vi "adam-analog-data-read.vi"(8 "error in (no error)":errorcluster, 9 "overwrite-command":string, 10 "current-buffer":string, 11 "VISA Refnum in":refnum<visa-resource-name>) -> (0 "error out":errorcluster, 1 "return count":u32, 2 "read buffer":string, 3 "VISA Refnum Out":refnum<visa-resource-name>, 5 "Bytes at Port":u32)   [LabVIEW 2024]
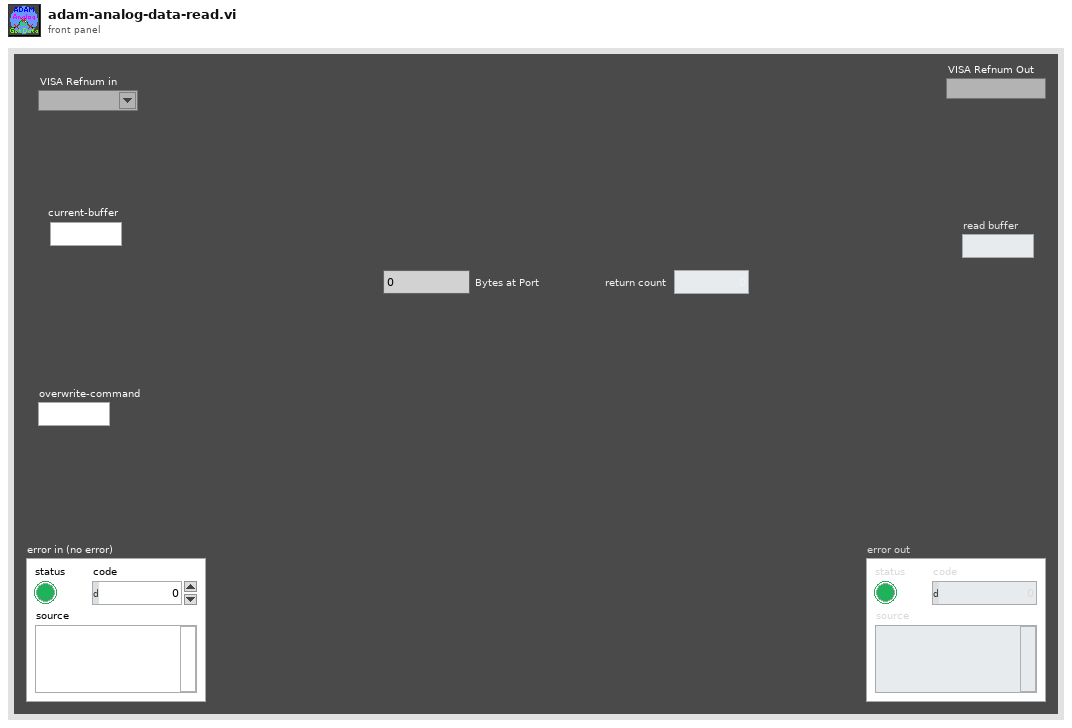
[diagram p1: front panel]
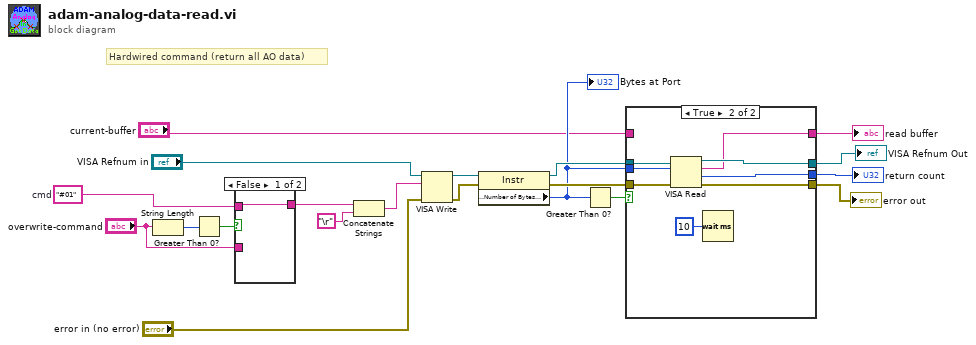
[diagram p0: block diagram]
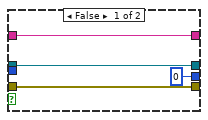
[diagram p3: hidden frame]
diagram:
  w12 = "#01"  # cmd
  # "Hardwired command (return all AO data)"
  n1 = String Length(string="overwrite-command") -> (length=w15:i32)
  n2 = Greater Than 0?(x=w15) -> (x > 0?=w14:bool)
  n3 = case shown="False" w14 {
    tunnel: "overwrite-command" -> [_ w22]
    tunnel: w12 -> [w21 _]
    tunnel: [w21 w22] -> w2
    frame False {
    }
    frame True {
    }
  }
  n4 = Concatenate Strings(w2, "\r") -> (w3:string)
  n5 = VISA Write(VISA resource name="VISA Refnum in", write buffer=w3, error in (no error)="error in (no error)") -> (VISA resource name out=w17:refnum<visa-resource-name>, error out=w19:errorcluster)  [unwired: 1 out]
  n6 = property class="Instr"(reference=w17, error in=w19) -> (reference out=w11:refnum<visa-resource-name>, error out=w10:errorcluster, "Serial Settings:Number of Bytes at Serial Port"=w8:u32)
  "Bytes at Port" <- w8
  n7 = Greater Than 0?(x=w8) -> (x > 0?=w20:bool)
  n8 = case shown="True" w20 {
    tunnel: w10 -> [w25 w33]
    tunnel: w11 -> [w26 w34]
    tunnel: [w26 w32] -> w6
    tunnel: [w25 w31] -> w9
    tunnel: [w24 w30] -> w7
    tunnel: w8 -> [_ w28]
    tunnel: "current-buffer" -> [w24 _]
    tunnel: [u32 0 ("return count") w27] -> w4
    frame False {
    }
    frame True {
      n9 = VISA Read(VISA resource name=w34, byte count=w28, error in (no error)=w33) -> (VISA resource name out=w32:refnum<visa-resource-name>, read buffer=w30:string, return count=w27:u32, error out=w31:errorcluster)
      n10 = Wait (ms)(milliseconds to wait=u32 10) -> ()  [unwired: 1 out]
    }
  }
  "error out" <- w9
  "read buffer" <- w7
  "VISA Refnum Out" <- w6
  "return count" <- w4
